vi "LoadDictionnaire.vi"(8 "error in (no error)":errorcluster, 11 "FichierDictionnaire":path) -> (0 "error out":errorcluster, 3 "Dictionnaire":T1)   [LabVIEW 2011]
uses:
  Dictionnaire.ctl
  CleValeur.ctl
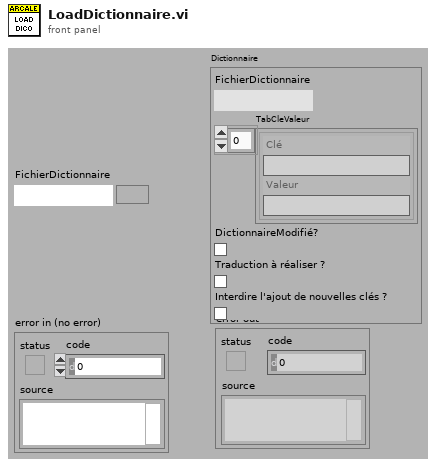
[diagram p1: front panel]
types:
  T1 = typedef "Dictionnaire.ctl" = cluster{"FichierDictionnaire":path, "TabCleValeur":T2[], "DictionnaireModifié?":bool, "Traduction à réaliser ?":bool, "Interdire l'ajout de nouvelles clés ?":bool}
  T2 = typedef "CleValeur.ctl" = cluster{"Clé":string, "Valeur":string}
  T3 = enum16{"open", "replace", "create", "open or create", "replace or create", "replace or create with confirmation"}
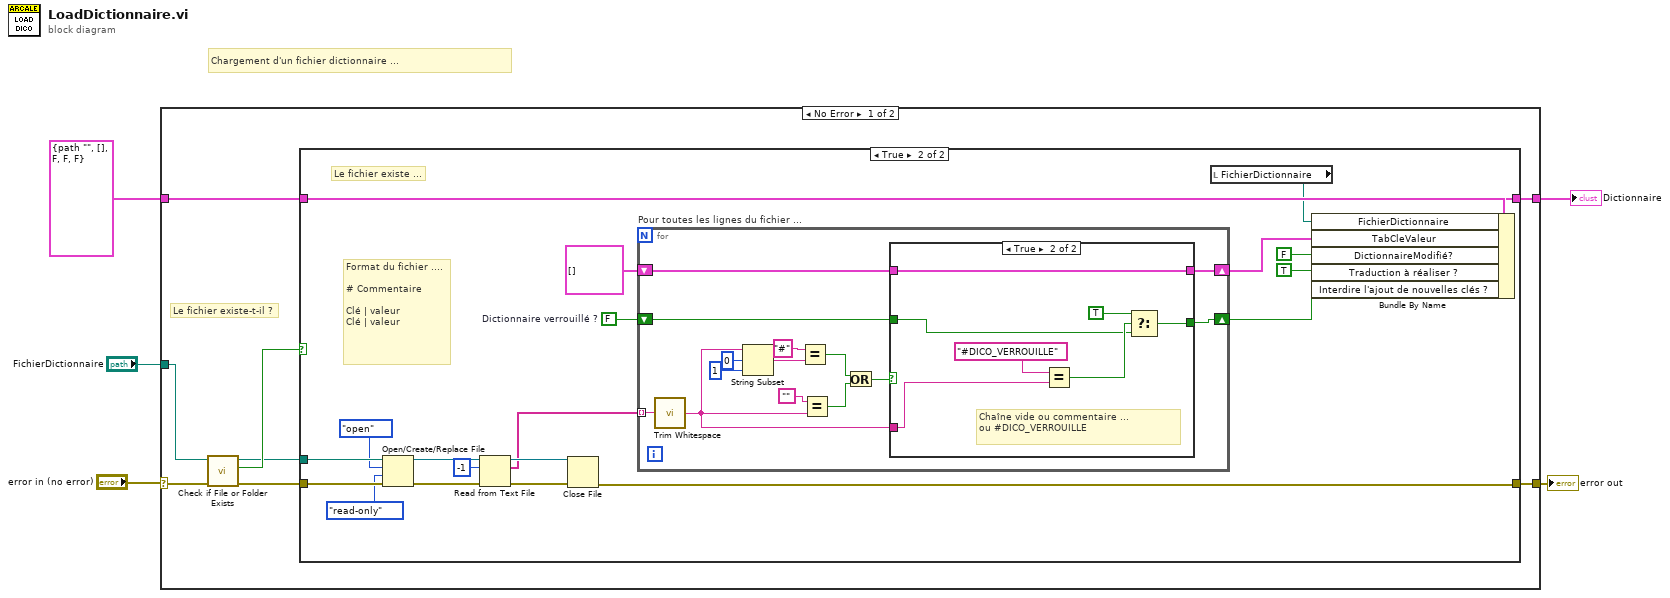
[diagram p0: block diagram]
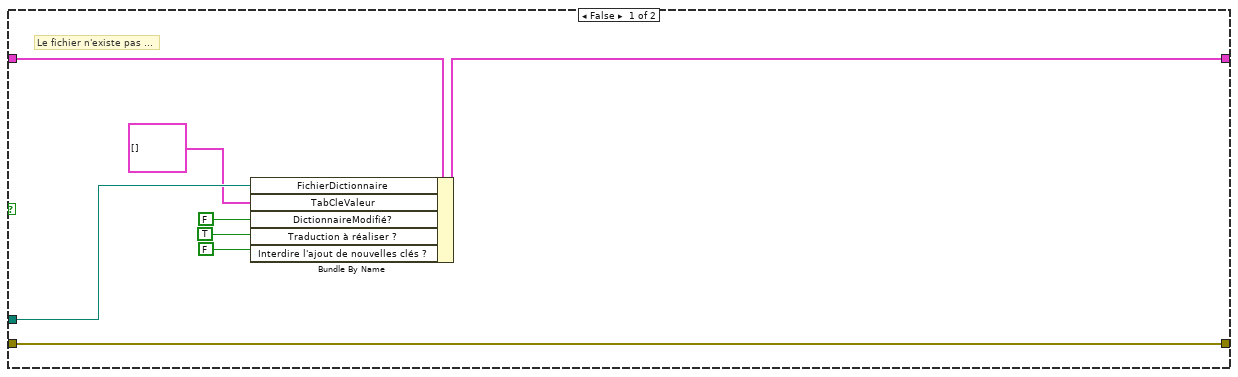
[diagram p2: hidden frame]
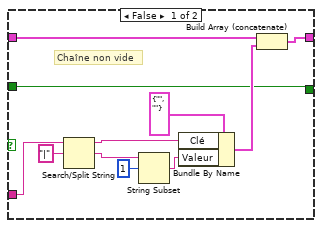
[diagram p3: hidden frame]
diagram:
  # "Chargement d'un fichier dictionnaire ..."
  n1 = case shown="No Error" "error in (no error)" {
    selector: "error in (no error)" -> [w13 w75]
    tunnel: "FichierDictionnaire" -> [w11 _]
    tunnel: [w6 w75] -> w3
    tunnel: T1 {"FichierDictionnaire"=path "", "TabCleValeur"=[], "DictionnaireModifié?"=FALSE, "Traduction à réaliser ?"=FALSE, "Interdire l'ajout de nouvelles clés ?"=FALSE} ("Dictionnaire") -> [w9 w74]
    tunnel: [w7 w74] -> w1
    frame No Error {
      # "Le fichier existe-t-il ?"
      n2 = call <vilib>:"Check if File or Folder Exists.vi"("error in (no error)"=w13, "path"=w11) -> ("error out"=w12:errorcluster, "file or folder exists?"=w10:bool, "dup path"=w8:path)  [unwired: 7 in]
      n3 = case shown="True" w10 {
        tunnel: w12 -> [w15 w41]
        tunnel: w9 -> [w21 w29]
        tunnel: w8 -> [w20 w40]
        tunnel: [w16 w28] -> w7
        tunnel: [w15 w31] -> w6
        frame False {
          # "Le fichier n'existe pas ..."
          n4 = Bundle By Name(cluster=w21, "FichierDictionnaire"=w20, "TabCleValeur"=T2[] [], "DictionnaireModifié?"=FALSE, "Traduction à réaliser ?"=TRUE, "Interdire l'ajout de nouvelles clés ?"=FALSE) -> (w16:T1)
        }
        frame True {
          w24 = FALSE  # Dictionnaire verrouillé ?
          # "Format du fichier ....\n\n# Commentaire\n\nClé | valeur\nClé | valeur"
          # "Le fichier existe ..."
          n5 = Open/Create/Replace File(file path (use dialog)=w40, error in=w41, operation (0:open)=T3."open", access (0:read/write)=enum16{"read/write", "read-only", "write-only"}."read-only") -> (refnum out=w36:refnum<file>, error out=w37:errorcluster)  [unwired: 2 in, 1 out]
          n6 = Read from Text File(file (use dialog)=w36, count=-1, error in=w37) -> (refnum out=w33:refnum<file>, text=w32:string[], error out=w34:errorcluster)  [unwired: 1 in, 1 out]
          n7 = Close File(refnum=w33, error in=w34) -> (error out=w31:errorcluster)  [unwired: 1 out]
          n8 = for "Pour toutes les lignes du fichier ..." {
            tunnel: w32 -> [w55] mode=indexing
            shift-right: [w45] -> w27
            shift-left: T2[] [] ("TabCleValeur") -> [w46]
            shift-right: [w42] -> w22
            shift-left: w24 -> [w43]
            n9 = call <vilib>:"Trim Whitespace.vi"("string"=w55) -> ("trimmed string"=w44:string)  [unwired: 1 in]
            n10 = String Subset(string=w44, offset (0)=0, length (rest)=1 ("length (rest)")) -> (substring=w52:string)
            n11 = Equal?(x="#", y=w52) -> (x = y?=w48:bool)
            n12 = Equal?(x="", y=w44) -> (x = y?=w49:bool)
            n13 = Or(x=w48, y=w49) -> (x .or. y?=w47:bool)
            n14 = case shown="True" w47 {
              tunnel: w46 -> [w66 w73]
              tunnel: [w65 w73] -> w45
              tunnel: w44 -> [w64 w72]
              tunnel: w43 -> [w56 w69]
              tunnel: [w56 w68] -> w42
              frame False {
                # "Chaîne non vide"
                n15 = Search/Split String(string=w64, search string/char (-)="|") -> (substring before match=w61:string, match + rest of string=w60:string)  [unwired: 1 in, 1 out]
                n16 = String Subset(string=w60, offset (0)=1) -> (substring=w58:string)  [unwired: 1 in]
                n17 = Bundle By Name(cluster=T2 {"Clé"="", "Valeur"=""} ("CléValeur"), "Clé"=w61, "Valeur"=w58) -> (w57:T2)
                n18 = Build Array (concatenate)(w66, w57) -> (w65:T2[])
              }
              frame True {
                # "Chaîne vide ou commentaire ...\nou #DICO_VERROUILLE"
                n19 = Equal?(x="#DICO_VERROUILLE", y=w72) -> (x = y?=w70:bool)
                n20 = Select(t=TRUE, s=w70, f=w69) -> (s? t:f=w68:bool)
              }
            }
          }
          n21 = local read "FichierDictionnaire"() -> (w23:path)
          n22 = Bundle By Name(cluster=w29, "FichierDictionnaire"=w23, "TabCleValeur"=w27, "DictionnaireModifié?"=FALSE, "Traduction à réaliser ?"=TRUE, "Interdire l'ajout de nouvelles clés ?"=w22) -> (w28:T1)
        }
      }
    }
    frame Error {
    }
  }
  "error out" <- w3
  "Dictionnaire" <- w1
